vi "N Channel N Samples - Manual Timestamp.vi"() -> ()   [LabVIEW 2026, in "synnax_clib.lvlib"]
uses:
  lvlib/synnax_clib.lvlib
  lvlib/typedefs/connection_config.ctl
  lvlib/classes/Client/Private/synnax channel retrieve keys Array.vi
  lvlib/classes/Writer/Private/synnax writer open Array.vi
  lvlib/classes/Writer/Private/Writes/I32/Write NCh NSamp (I32).vi
  lvlib/classes/Synnax Writer.lvclass
  lvlib/classes/Client/Synnax Client.lvclass
panel:
  in  "Channels":string[](array[numeric])=["my_i32_idx", "my_i32_ch1", "my_i32_ch2", "my_i32_ch3", "my_i32_ch4"]
  in  "Stop":bool
  out "error out":errorcluster
  in  "Connection Config":T1={"host"="localhost", "port"=9090, "username"="synnax", "password"="seldon"}
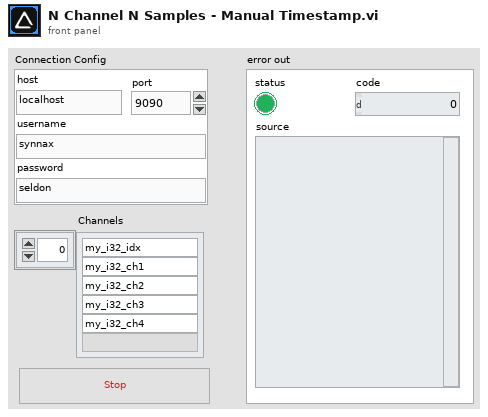
[diagram p1: front panel]
types:
  T1 = typedef "synnax_clib.lvlib/connection_config.ctl" = cluster{"host":string, "port":u16, "username":string, "password":string}
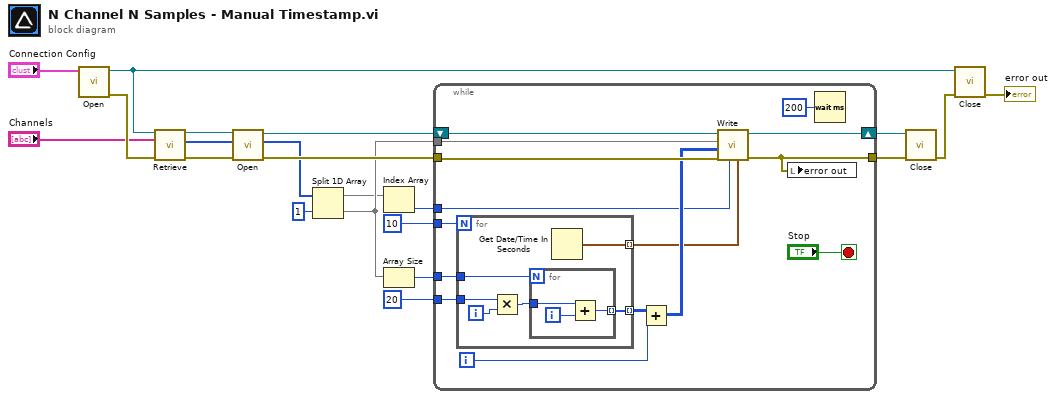
[diagram p0: block diagram]
diagram:
  n1 = call "Open.vi"("Connection Config"="Connection Config") -> ("error out"=w16:errorcluster, "Synnax Client out"=w18:refnum<class "Synnax Client.lvclass">)  [unwired: 9 in]
  n2 = call-poly "Retrieve.vi"("Synnax Client in"=w18, "channel names"="Channels", "error in"=w16) -> ("Synnax Client out"=w12:refnum<class "Synnax Client.lvclass">, "channel keys"=w10:u32[], "error out"=w20:errorcluster)  [unwired: 8 in, 2 out]
  n3 = call-poly "Open.vi"("error in"=w20, "channels in"=w10, "Synnax Client in"=w12) -> ("error out"=w13:errorcluster, "channels out"=w4:u32[], "writer out"=w15:refnum<class "Synnax Writer.lvclass">)  [unwired: 6 in]
  n4 = Split 1D Array(array=w4, index=1) -> (first subarray=w2:u32[], second subarray=w3:u32[])
  n5 = Index Array(array=w2) -> (element=w1:u32)  [unwired: 1 in]
  n6 = Array Size(array=w3) -> (size(s)=w8:i32)
  n7 = while {
    shift-right: [w35] -> w14
    shift-left: w15 -> [w36]
    tunnel: w13 -> [w34]
    tunnel: [w31] -> w21
    tunnel: w3 -> [w29]
    tunnel: w8 -> [w22]
    tunnel: 10 -> [w23]
    tunnel: 20 -> [w26]
    tunnel: w1 -> [w25]
    i -> [w27]
    stop <- "Stop" stop-if-true
    n8 = for {
      N: w23 -> [_]
      tunnel: [w42] -> w32 mode=indexing
      tunnel: w22 -> [w38]
      tunnel: w26 -> [w39]
      tunnel: [w37] -> w24 mode=indexing
      i -> [w40]
      n9 = Multiply(x=w39, y=w40) -> (x*y=w41:i32)
      n10 = for {
        N: w38 -> [_]
        tunnel: [w43] -> w42 mode=indexing
        tunnel: w41 -> [w45]
        i -> [w44]
        n11 = Add(x=w45, y=w44) -> (x+y=w43:i32)
      }
      n12 = Get Date/Time In Seconds() -> (seconds since 1Jan1904=w37:timestamp)
    }
    n13 = Add(x=w32, y=w27) -> (x+y=w28:i32[][])
    n14 = call-poly "Write.vi"("timestamps"=w24, "index_channel"=w25, "error in"=w34, "data"=w28, "channels"=w29, "Writer"=w36) -> ("error out"=w31:errorcluster, "Writer Out"=w35:refnum<class "Synnax Writer.lvclass">)  [unwired: 4 in]
    n15 = local write "error out"(w31) -> ()
    n16 = Wait (ms)(milliseconds to wait=u32 200) -> ()  [unwired: 1 out]
  }
  n17 = call "Close.vi"("error in"=w21, "writer"=w14) -> ("error out"=w17:errorcluster)  [unwired: 9 in]
  n18 = call "Close.vi"("error in"=w17, "Synnax Client in"=w18) -> ("error out"=→"error out":errorcluster)  [unwired: 9 in]
